vi "RunPositionNet.vi"(10 "Input Vector":dbl[](array[numeric]), 11 "Weights":cluster{"A - B":T1}[](array[cluster])) -> (3 "Output Vector":dbl[](array[numeric]))   [LabVIEW 2016]
uses:
  <vilib>/Analysis/Matrix/Datatypes/RealMatrix.ctl
  <vilib>/Analysis/baseanly.llb/A x Vector.vi
  <vilib>/Analysis/NI_AALBase.lvlib
  <vilib>/Analysis/Matrix/NI_Matrix.lvlib
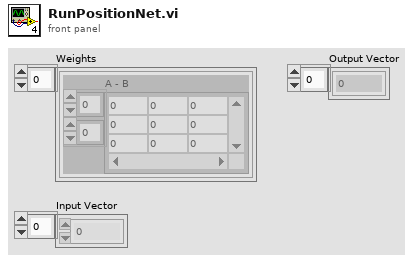
[diagram p1: front panel]
types:
  T1 = typedef "NI_Matrix.lvlib/RealMatrix.ctl" = dbl[][]
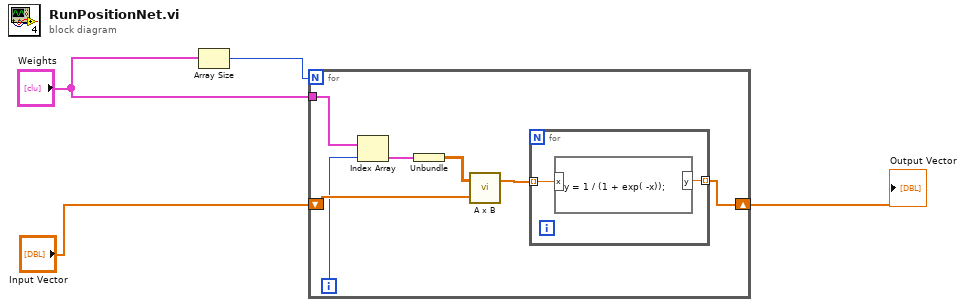
[diagram p0: block diagram]
diagram:
  n1 = Array Size(array="Weights") -> (size(s)=w1:i32)
  n2 = for {
    N: w1 -> [_]
    tunnel: "Weights" -> [w11]
    shift-right: [w5] -> w3
    shift-left: "Input Vector" -> [w9]
    i -> [w7]
    n3 = Index Array(array=w11, index=w7) -> (element=w10:cluster{"A - B":T1})
    n4 = Unbundle(w10) -> ("A - B"=w8:T1)
    n5 = call-poly <vilib>:"A x B.vi"("Vector"=w9, "A"=w8) -> ("A x Vector"=w6:dbl[])  [unwired: 1 out]
    n6 = for {
      tunnel: w6 -> [w13] mode=indexing
      tunnel: [w12] -> w5 mode=indexing
      n7 = formula code="y = 1 / (1 + exp( -x));"("x"=w13) -> ("y"=w12:dbl)
    }
  }
  "Output Vector" <- w3
